vi "B-Scan (Timed) DVR - MultiChannel.vi"(9 "Scan definition":T2={"Max Scan Length"=0, "Update Rate"=1000, "Direction"=enum."Forwards"} {"Update Rate" format="%#_6f"; "Max Scan Length" format="%#_6f"}, 10 "scan data info":T4 {"Error Message" format="%04x"; "Message Header" format="%04x"; "IP"."MIP location" format="%#.0f"; "IP"."Location" format="%#.0f"; "PRF" format="%.0fHz"}, 11 "Test #":i32=1 min=1 max=1279) -> (0 "Update Display?":bool, 1 "B-Scan In Progress?":bool, 2 "B-Scan Finished?":bool, 3 "data value reference":refnum<data-value>, 4 "B-Scan Index":i32)   [LabVIEW 2026, in "MicroPulse_Driver.lvlib"]
uses:
  MicroPulse_Driver.lvlib
  Data/Datatypes/MP - scan data info.ctl
  Data/Datatypes/MP - data output format.ctl
  Data/Datatypes/MP - retain scan.ctl
  Data/Datatypes/MP - axis positions (LLC).ctl
  Data/Datatypes/MP - fly scan range (timed).ctl
  Data/Datatypes/MP - inspection direction.ctl
  Low Level/FGV - B-Scan Active - Action [Enum].ctl
  <instrlib>/Micropulse/Micropulse.lvlib
panel:
  in  "X Scan definition":T1={"Max X Scan Length"=0, "Indexing\nResolution"=1000} {"Indexing\nResolution" format="%#_6f"; "Max X Scan Length" format="%#_6f"}
  # "X-Scan Index"
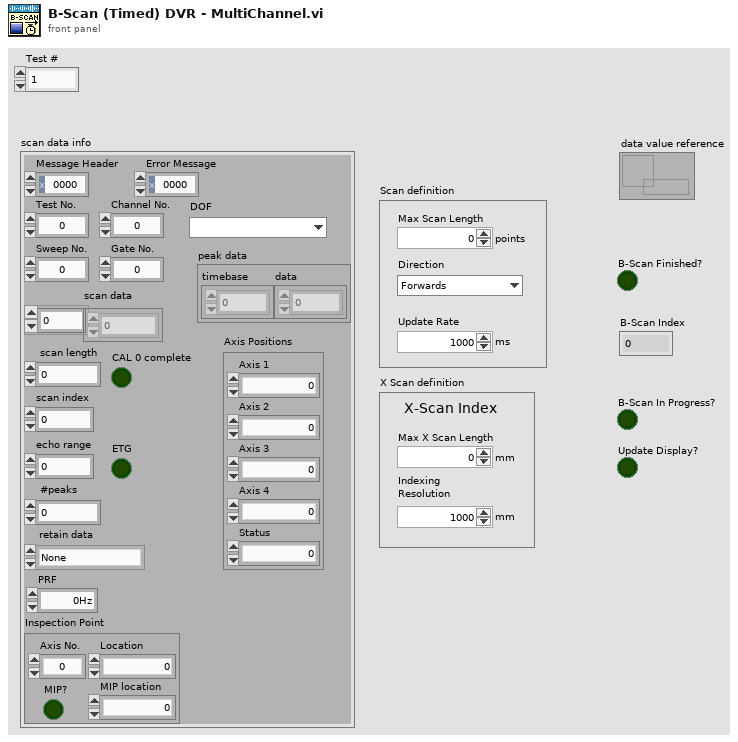
[diagram p1: front panel]
types:
  T1 = cluster{"Max X Scan Length":i32, "Indexing\nResolution":i32}
  T2 = typedef "Micropulse.lvlib/MP - fly scan range (timed).ctl" = cluster{"Max Scan Length":i32, "Update Rate":i32, "Direction":T3}
  T3 = typedef "Micropulse.lvlib/MP - inspection direction.ctl" = enum16{"Forwards", "Backwards"}
  T4 = typedef "Micropulse.lvlib/MP - scan data info.ctl" = cluster{"Message Header":u16, "Error Message":u16, "Test No.":u32, "Channel No.":u8, "Sweep No.":u32, "Gate No.":u32, "DOF":T5, "retain data":T6, "scan data":u16[], "scan length":i32, "scan index":i32, "peak data":cluster{"timebase":u16[], "data":u16[]}, "#peaks":i32, "PRF":dbl, "IP":cluster{"Axis No.":u8, "Location":u32, "MIP location":u32, "MIP?":bool}, "echo range":u16, "ETG":bool, "CAL 0 complete":bool, "Axis Positions":T7}
  T5 = typedef "Micropulse.lvlib/MP - data output format.ctl" = enum16{"", "8-bit Mode", "10-bit Mode", "12-bit Mode", "16-bit Mode", "8-bit Log Mode", "12-bit Packed Mode"}
  T6 = typedef "Micropulse.lvlib/MP - retain scan.ctl" = enum16{"None", "Ascan", "Peaks"}
  T7 = typedef "Micropulse.lvlib/MP - axis positions (LLC).ctl" = cluster{"Axis 1":u32, "Axis 2":u32, "Axis 3":u32, "Axis 4":u32, "Status":u8}
  T8 = typedef "MicroPulse_Driver.lvlib/FGV - B-Scan Active - Action [Enum].ctl" = enum16{"Read", "Read & Reset Start Flag", "Start B-Scan", "B-Scan Finished"}
  T9 = cluster{"Lowest location":i32, "Highest location":i32}
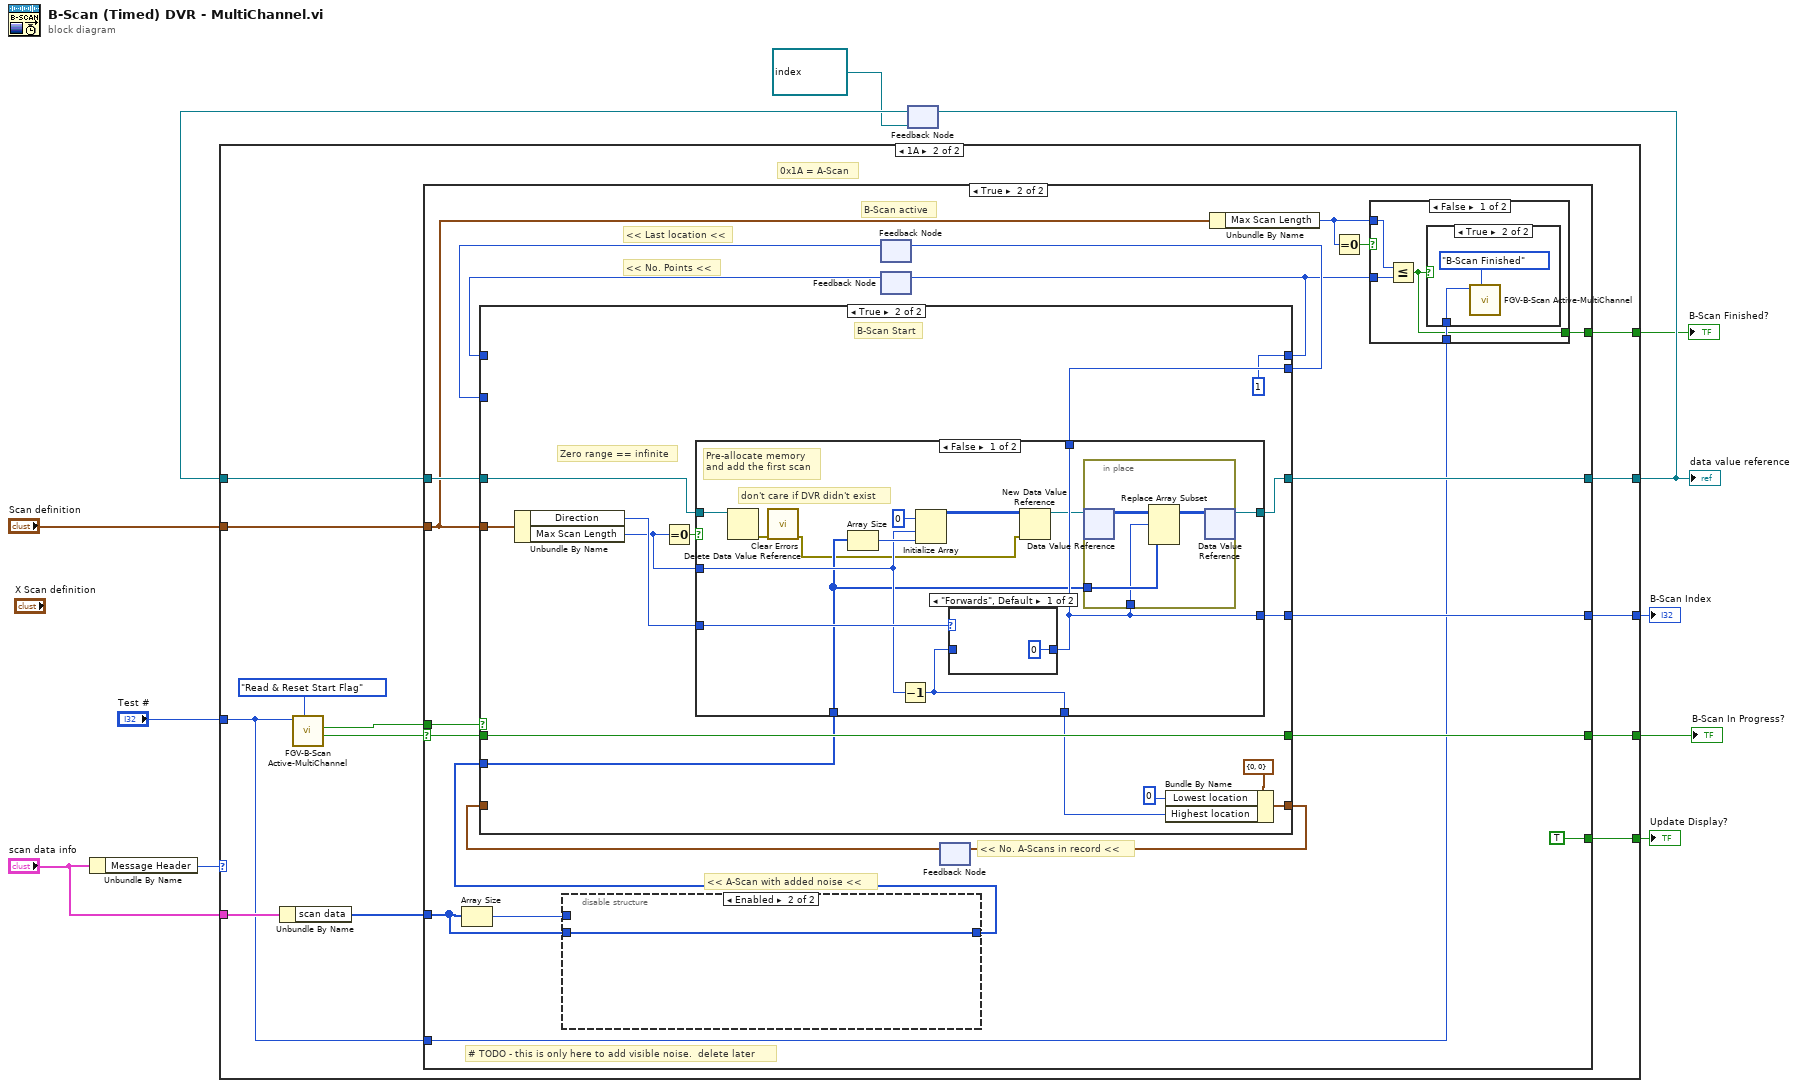
[diagram p0: block diagram]
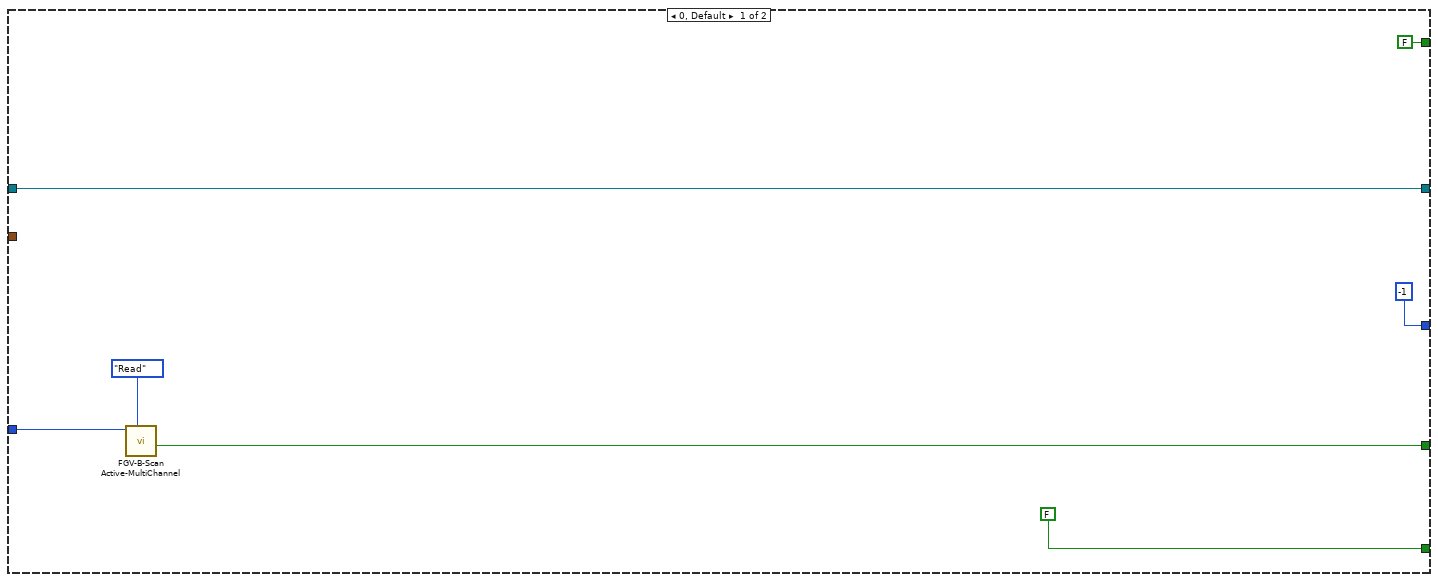
[diagram p2: hidden frame]
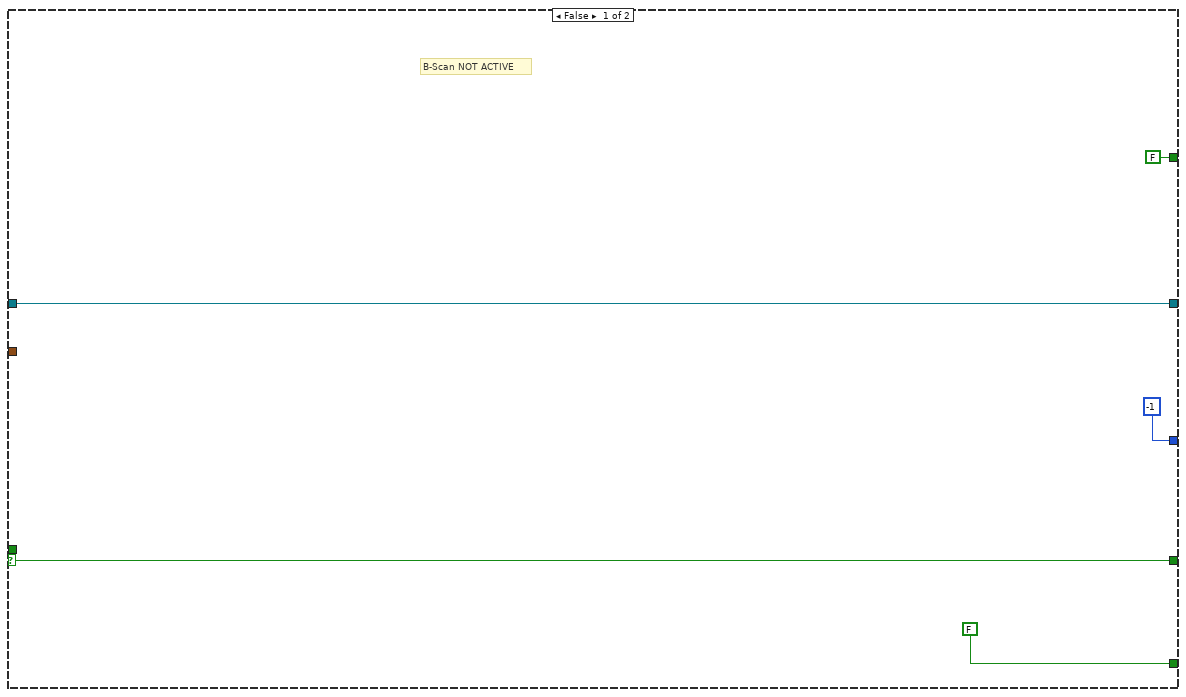
[diagram p3: hidden frame]
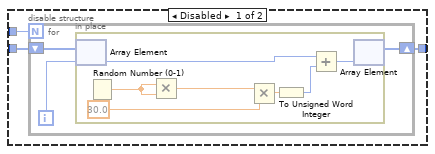
[diagram p4: hidden frame]
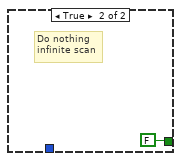
[diagram p6: hidden frame]
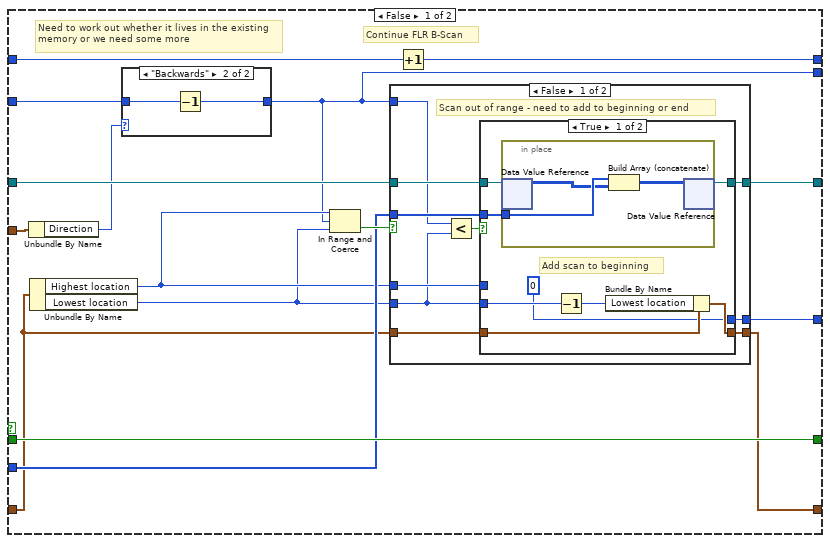
[diagram p7: hidden frame]
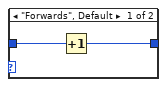
[diagram p8: hidden frame]
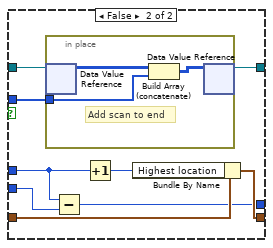
[diagram p9: hidden frame]
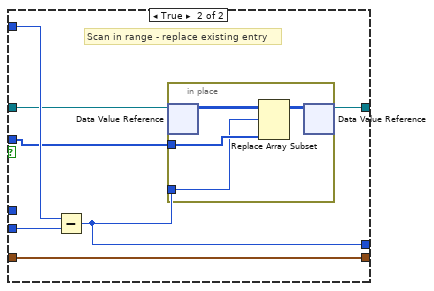
[diagram p10: hidden frame]
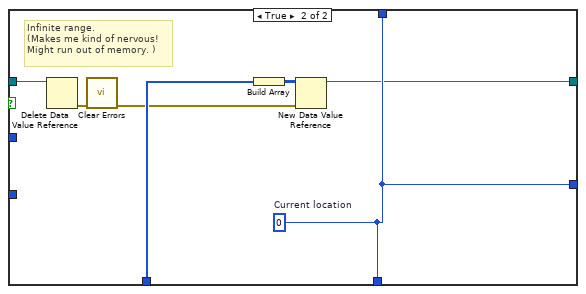
[diagram p12: hidden frame]
diagram:
  n1 = Unbundle By Name("scan data info") -> ("Message Header"=w11:u16)
  n2 = feedback #1(refnum<data-value> refnum ("data value reference")) -> (w8:refnum<data-value>)
  n3 = case shown="1A" w11 {
    tunnel: "scan data info" -> [_ w31]
    tunnel: "Scan definition" -> [_ w25]
    tunnel: [w18 w29] -> w9
    tunnel: w8 -> [w18 w28]
    tunnel: [w15 w27] -> w7
    tunnel: [FALSE w26] -> w6
    tunnel: [-1 ("Current location") w21] -> w4
    tunnel: "Test #" -> [w13 w20]
    tunnel: [FALSE w19] -> w1
    frame 0, Default {
      n4 = call "FGV-B-Scan Active-MultiChannel.vi"("Action"=FGV_-_B-Scan_Active_-_Action_[Enum]."Read", "Test #"=w13) -> ("B-Scan In Progress?"=w15:bool)  [unwired: 7 in, 2 out]
    }
    frame 26 {
      # "0x1A = A-Scan"
      n5 = Unbundle By Name(w31) -> ("scan data"=w30:u16[])
      n6 = call "FGV-B-Scan Active-MultiChannel.vi"("Action"=FGV_-_B-Scan_Active_-_Action_[Enum]."Read & Reset Start Flag", "Test #"=w20) -> ("B-Scan In Progress?"=w22:bool, "B-Scan Start?"=w23:bool)  [unwired: 7 in, 1 out]
      n7 = case shown="True" w22 {
        selector: w22 -> [w35 w53]
        tunnel: w23 -> [_ w56]
        tunnel: w28 -> [w36 w57]
        tunnel: [w36 w50] -> w29
        tunnel: w30 -> [_ w49]
        tunnel: w25 -> [_ w43]
        tunnel: [w35 w54] -> w27
        tunnel: [FALSE TRUE] -> w26
        tunnel: [-1 ("Current location") w39] -> w21
        tunnel: w20 -> [_ w38]
        tunnel: [FALSE w37] -> w19
        frame False {
          # "B-Scan NOT ACTIVE"
        }
        frame True {
          # "<< No. Points <<"
          # "<< Last location <<"
          # "<< A-Scan with added noise <<"
          # "B-Scan active"
          # "<< No. A-Scans in record <<"
          # "# TODO - this is only here to add visible noise.  delete later"
          n8 = Array Size(array=w49) -> (size(s)=w51:i32)
          n9 = disable-structure shown="Enabled" {
            disable-tunnel: w51 -> [w60 _]
            disable-tunnel: w49 -> [w59 w71]
            disable-tunnel: [w58 w71] -> w48
            frame Disabled {
              n10 = for {
                N: w60 -> [_]
                shift-right: [w61] -> w58
                shift-left: w59 -> [w63]
                i -> [w62]
                n11 = in-place {
                  n12 = in-place-array #2(w63, w62) -> (w67:u16)
                  n13 = Random Number (0-1)() -> (number: 0 to 1=w64:dbl)
                  n14 = Multiply(x=w64, y=w64) -> (x*y=w65:dbl)
                  n15 = Multiply(x=w65, y=30.0) -> (x*y=w69:dbl)
                  n16 = To Unsigned Word Integer(number=w69) -> (unsigned 16bit integer=w68:u16)
                  n17 = Add(x=w67, y=w68) -> (x+y=w66:u16)
                  n18 = in-place-array #2(w66) -> (w61:u16[])  [unwired: 1 out]
                }
              }
            }
            frame Enabled {
            }
          }
          n19 = feedback #3() -> (w45:i32)  [unwired: 1 in]
          n20 = feedback #4() -> (w44:i32)  [unwired: 1 in]
          n21 = feedback #5() -> (w55:T9)  [unwired: 1 in]
          n22 = case shown="True" w56 {
            tunnel: w57 -> [w94 w143]
            tunnel: [w92 w157] -> w50
            tunnel: w43 -> [w85 w156]
            tunnel: w45 -> [w83 _]
            tunnel: w55 -> [w87 _]
            tunnel: [w93 w155] -> w54
            tunnel: w53 -> [w93 w155]
            tunnel: w48 -> [w90 w154]
            tunnel: [w86 w152] -> w47
            tunnel: [w82 w146] -> w46
            tunnel: [w80 1 ("Current location")] -> w40
            tunnel: w44 -> [w81 _]
            tunnel: [w79 w144] -> w39
            frame False {
              # "Continue FLR B-Scan"
              # "Need to work out whether it lives in the existing memory or we need some more"
              n23 = Unbundle By Name(w85) -> ("Direction"=w84:T3)
              n24 = Unbundle By Name(w87) -> ("Highest location"=w89:i32, "Lowest location"=w88:i32)
              n25 = case shown="\"Backwards\"" w84 {
                tunnel: w83 -> [w96 w98]
                tunnel: [w95 w97] -> w82
                frame "Forwards", Default {
                  n26 = Increment(x=w96) -> (x+1=w95:i32)
                }
                frame "Backwards" {
                  n27 = Decrement(x=w98) -> (x-1=w97:i32)
                }
              }
              n28 = In Range and Coerce(upper limit=w89, x=w82, lower limit=w88) -> (In Range?=w91:bool)  [unwired: 1 out]
              n29 = case shown="False" w91 {
                tunnel: w94 -> [w108 w134]
                tunnel: [w107 w135] -> w92
                tunnel: w82 -> [w105 w138]
                tunnel: w90 -> [w106 w132]
                tunnel: w89 -> [w103 _]
                tunnel: w88 -> [w100 w136]
                tunnel: w87 -> [w102 w137]
                tunnel: [w101 w137] -> w86
                tunnel: [w99 w133] -> w79
                frame False {
                  # "Scan out of range - need to add to beginning or end"
                  n30 = Less?(x=w105, y=w100) -> (x < y?=w104:bool)
                  n31 = case shown="True" w104 {
                    tunnel: w108 -> [w110 w122]
                    tunnel: [w111 w120] -> w107
                    tunnel: w106 -> [w109 w121]
                    tunnel: w103 -> [_ w125]
                    tunnel: w100 -> [w115 w124]
                    tunnel: w102 -> [w116 w128]
                    tunnel: [w113 w126] -> w101
                    tunnel: [0 w123] -> w99
                    frame True {
                      # "Add scan to beginning"
                      n32 = in-place {
                        in-place-border: w109 -> [w119]
                        n33 = in-place-dvr #6(w110) -> (w118:u16[][])  [unwired: 1 out]
                        n34 = Build Array (concatenate)(w119, w118) -> (w117:u16[][])
                        n35 = in-place-dvr #6(w117) -> (w111:refnum<data-value>)  [unwired: 1 out]
                      }
                      n36 = Decrement(x=w115) -> (x-1=w114:i32)
                      n37 = Bundle By Name(cluster=w116, "Lowest location"=w114) -> (w113:T9)
                    }
                    frame False {
                      n38 = in-place {
                        in-place-border: w121 -> [w131]
                        # "Add scan to end"
                        n39 = in-place-dvr #7(w122) -> (w129:u16[][])  [unwired: 1 out]
                        n40 = Build Array (concatenate)(w129, w131) -> (w130:u16[][])
                        n41 = in-place-dvr #7(w130) -> (w120:refnum<data-value>)  [unwired: 1 out]
                      }
                      n42 = Subtract(x=w125, y=w124) -> (x-y=w123:i32)
                      n43 = Increment(x=w125) -> (x+1=w127:i32)
                      n44 = Bundle By Name(cluster=w128, "Highest location"=w127) -> (w126:T9)
                    }
                  }
                }
                frame True {
                  # "Scan in range - replace existing entry"
                  n45 = Subtract(x=w138, y=w136) -> (x-y=w133:i32)
                  n46 = in-place {
                    in-place-border: w132 -> [w142]
                    in-place-border: w133 -> [w141]
                    n47 = in-place-dvr #8(w134) -> (w139:u16[][])  [unwired: 1 out]
                    n48 = Replace Array Subset(array=w139, new element=w142, index (row)=w141) -> (w140:u16[][])  [unwired: 1 in]
                    n49 = in-place-dvr #8(w140) -> (w135:refnum<data-value>)  [unwired: 1 out]
                  }
                }
              }
              n50 = Increment(x=w81) -> (x+1=w80:i32)
            }
            frame True {
              # "Zero range == infinite"
              # "B-Scan Start"
              n51 = Unbundle By Name(w156) -> ("Direction"=w151:T3, "Max Scan Length"=w148:i32)
              n52 = Equal To 0?(x=w148) -> (x = 0?=w149:bool)
              n53 = case shown="False" w149 {
                tunnel: [w160 w177] -> w157
                tunnel: w148 -> [w167 _]
                tunnel: w154 -> [w159 w183]
                tunnel: w151 -> [w168 _]
                tunnel: [w166 w182] -> w150
                tunnel: [w163 w182] -> w146
                tunnel: [w163 w182] -> w144
                tunnel: w143 -> [w164 w179]
                frame False {
                  # "don't care if DVR didn't exist"
                  # "Pre-allocate memory\nand add the first scan"
                  n54 = Delete Data Value Reference(data value reference=w164) -> (error out=w165:errorcluster)  [unwired: 1 in, 1 out]
                  n55 = call <vilib>:"Clear Errors.vi"("error in (no error)"=w165) -> ("error out"=w158:errorcluster)  [unwired: 5 in, 1 out]
                  n56 = Array Size(array=w159) -> (size(s)=w169:i32)
                  n57 = Decrement(x=w167) -> (x-1=w166:i32)
                  n58 = Initialize Array(u16 0 ("index"), w167, w169) -> (w161:u16[][])
                  n59 = case shown="\"Forwards\", Default" w168 {
                    tunnel: w166 -> [_ w176]
                    tunnel: [0 w176] -> w163
                    frame "Forwards", Default {
                    }
                    frame "Backwards" {
                    }
                  }
                  n60 = New Data Value Reference(data value=w161, error in=w158) -> (data value reference=w162:refnum<data-value>)  [unwired: 1 out]
                  n61 = in-place {
                    in-place-border: w159 -> [w174]
                    in-place-border: w163 -> [w173]
                    n62 = in-place-dvr #9(w162) -> (w172:u16[][])  [unwired: 1 out]
                    n63 = Replace Array Subset(array=w172, new element=w174, index (row)=w173) -> (w171:u16[][])  [unwired: 1 in]
                    n64 = in-place-dvr #9(w171) -> (w160:refnum<data-value>)  [unwired: 1 out]
                  }
                }
                frame True {
                  w182 = 0  # Current location
                  # "Infinite range.\n(Makes me kind of nervous!\nMight run out of memory. )"
                  n65 = Delete Data Value Reference(data value reference=w179) -> (error out=w180:errorcluster)  [unwired: 1 in, 1 out]
                  n66 = call <vilib>:"Clear Errors.vi"("error in (no error)"=w180) -> ("error out"=w181:errorcluster)  [unwired: 5 in, 1 out]
                  n67 = Build Array(w183) -> (w178:u16[][])
                  n68 = New Data Value Reference(data value=w178, error in=w181) -> (data value reference=w177:refnum<data-value>)  [unwired: 1 out]
                }
              }
              n69 = Bundle By Name(cluster=T9 {"Lowest location"=0, "Highest location"=0} ("input cluster"), "Lowest location"=0, "Highest location"=w150) -> (w152:T9)
            }
          }
          n70 = feedback-in #3(w46) -> ()
          n71 = feedback-in #4(w40) -> ()
          n72 = feedback-in #5(w47) -> ()
          n73 = Unbundle By Name(w43) -> ("Max Scan Length"=w41:i32)
          n74 = Equal To 0?(x=w41) -> (x = 0?=w42:bool)
          n75 = case shown="False" w42 {
            tunnel: w41 -> [w74 _]
            tunnel: w40 -> [w75 _]
            tunnel: w38 -> [w73 _]
            tunnel: [w72 FALSE] -> w37
            frame False {
              n76 = Less Or Equal?(x=w74, y=w75) -> (x <= y?=w72:bool)
              n77 = case shown="True" w72 {
                tunnel: w73 -> [_ w76]
                frame False {
                }
                frame True {
                  n78 = call "FGV-B-Scan Active-MultiChannel.vi"("Action"=FGV_-_B-Scan_Active_-_Action_[Enum]."B-Scan Finished", "Test #"=w76) -> ()  [unwired: 7 in, 3 out]
                }
              }
            }
            frame True {
              # "Do nothing\ninfinite scan"
            }
          }
        }
      }
    }
  }
  "data value reference" <- w9
  "Update Display?" <- w6
  "B-Scan In Progress?" <- w7
  "B-Scan Index" <- w4
  "B-Scan Finished?" <- w1
  n79 = feedback-in #1(w9) -> ()
